vi "Mathematical Model Air Heater.vi"(1 "Model Parameters":T1={"K [C/V]"=0.0, "T_delay [s]"=1.0, "T_env [Deg C]"=0.0, "T initial [Deg C]"=0.0, "T [s]"=0.0}, 2 "u [V]":dbl) -> (0 "T_out [deg C]":dbl)   [LabVIEW 2022 SP3]
uses:
  <vilib>/Simulation/Implementation/XNodeFramework/SimXNode/SimX.xnode
  <vilib>/Simulation/ContinuousLinear/Implementation/NILVSim Integrator new.llb/SIM Integrator (scalar).vi
  <vilib>/Simulation/ContinuousLinear/Implementation/NILVSim Transport Delay.llb/SIM Transport Delay Indirect (scalar).vi
  <vilib>/Simulation/Implementation/Shared/SIMSCR Execution Mode.ctl
  <vilib>/Simulation/Scripting/Companion Diagram/SimConfigNode/SimDog.xnode
  <vilib>/Simulation/Implementation/Shared/SIM Bundle Sim Info.vi
  <vilib>/Simulation/Implementation/Shared/SIM Unbundle Sim Info.vi
  <vilib>/Simulation/Implementation/Shared/SIM SimErrorHandler.vi
  <vilib>/Simulation/Implementation/Shared/NILVSim_FinalizeModel.vi
  <vilib>/Simulation/Implementation/Shared/NILVSim_GetModelError.vi
  <vilib>/Simulation/Implementation/Shared/NILVSim_Initialize.vi
  <vilib>/Simulation/Utility/Implementation/NILVSim Get Time and IsAcceptedStep.vi
  <vilib>/Simulation/Implementation/Shared/NILVSim_Manager.vi
  <vilib>/Simulation/Implementation/Shared/NI_SIM_Implementation.lvlib
  <vilib>/Simulation/Implementation/Shared/NILVSIM_BeginStep.vi
  <vilib>/Simulation/Param Hierarchy/Typedefs/SIMPH Param Control Actions.ctl
  <vilib>/Simulation/Implementation/Shared/NILVSim_ParamChanged.vi
  <vilib>/Utility/error.llb/Clear Errors.vi
  <vilib>/Simulation/Implementation/Shared/SIMSH Read Queue.vi
  <vilib>/Simulation/ContinuousLinear/Implementation/NILVSim Integrator new.llb/SIM Integrator distributor (scalar).vi
  <vilib>/Simulation/ContinuousLinear/Implementation/NILVSim Integrator new.llb/SIM Integrator collector (scalar).vi
  <vilib>/Simulation/Implementation/Shared/SIM limit type.ctl
  <vilib>/Simulation/ContinuousLinear/Implementation/NILVSim Transport Delay.llb/SIM Transport Delay Distributor (scalar).vi
  <vilib>/Simulation/ContinuousLinear/Implementation/NILVSim Transport Delay.llb/SIM Transport Delay Collector (scalar).vi
  <vilib>/Simulation/Scripting/Companion Diagram/SimConfigNode/_simSolvers.ctl
  <vilib>/Simulation/Scripting/Companion Diagram/SimConfigNode/SimParams.ctl
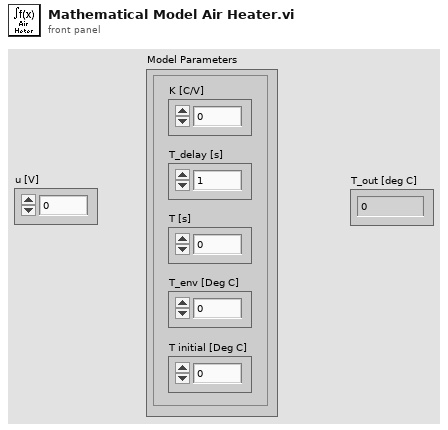
[diagram p1: front panel]
types:
  T1 = cluster{"K [C/V]":dbl, "T_delay [s]":dbl, "T_env [Deg C]":dbl, "T initial [Deg C]":dbl, "T [s]":dbl}
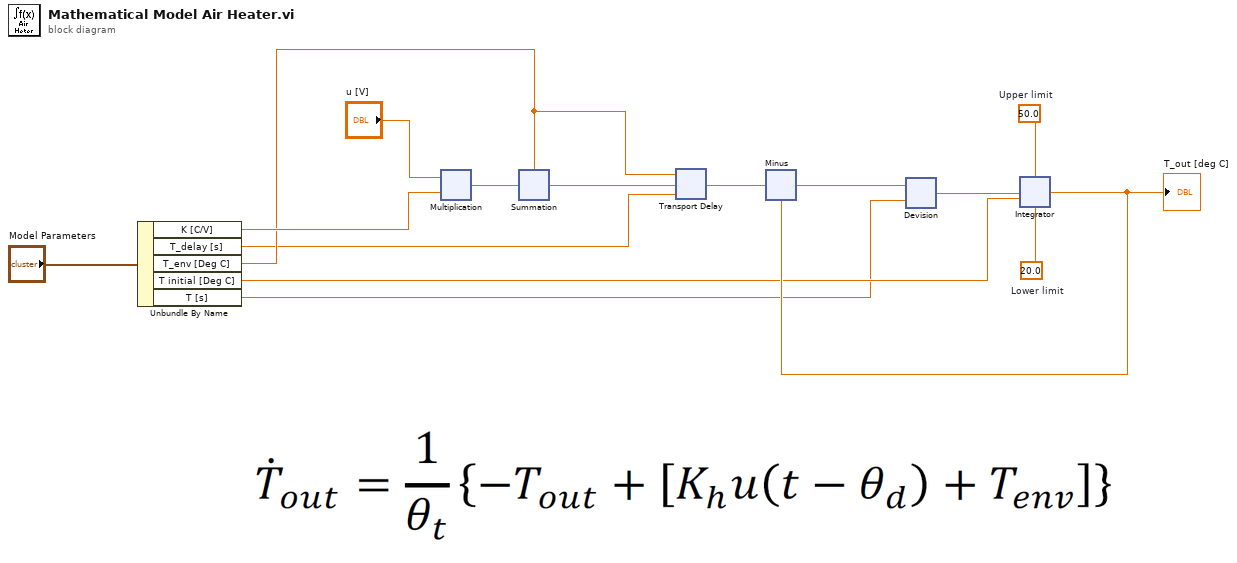
[diagram p0: block diagram]
diagram:
  w8 = 50.0  # Upper limit
  w9 = 20.0  # Lower limit
  n1 = Unbundle By Name("Model Parameters") -> ("K [C/V]"=w5:dbl, "T_delay [s]"=w3:dbl, "T_env [Deg C]"=w4:dbl, "T initial [Deg C]"=w2:dbl, "T [s]"=w1:dbl)
  n2 = xnode "Multiplication"("Operand1"="u [V]", "Operand2"=w5) -> ("Result"=w14:dbl)
  n3 = xnode "Summation"("Operand1"=w4, "Operand2"=w14) -> ("Result"=w13:dbl)
  n4 = xnode "Transport Delay"("initial condition"=w4, "input"=w13, "delay (s)"=w3) -> ("output"=w12:dbl)  [unwired: 2 in]
  n5 = xnode "Minus"("Operand1"=w12, "Operand2"=w7) -> ("Result"=w11:dbl)
  n6 = xnode "Devision"("Operand1"=w11, "Operand2"=w1) -> ("Result"=w10:dbl)
  n7 = xnode "Integrator"("upper limit"=w8, "input"=w10, "initial condition"=w2, "lower limit"=w9) -> ("output"=w7:dbl)  [unwired: 6 in, 2 out]
  "T_out [deg C]" <- w7
